vi "ScreenShots_Main_VIs.vi"(8 "error in":errorcluster, 9 "Bild Auswahl":T1[](array[typedef]), 10 "filename":string[](array[string]), 11 "Screenshots Pfad":path) -> (0 "error out":errorcluster, 3 "Screenshots Pfad out":path caption="Screenshots Pfad")   [LabVIEW 2020, in "Backup.lvlib"]
uses:
  Backup.lvlib
  Bildwechsel/Bild-Auswahl.ctl
  Bildwechsel/Bildwechsel.lvlib
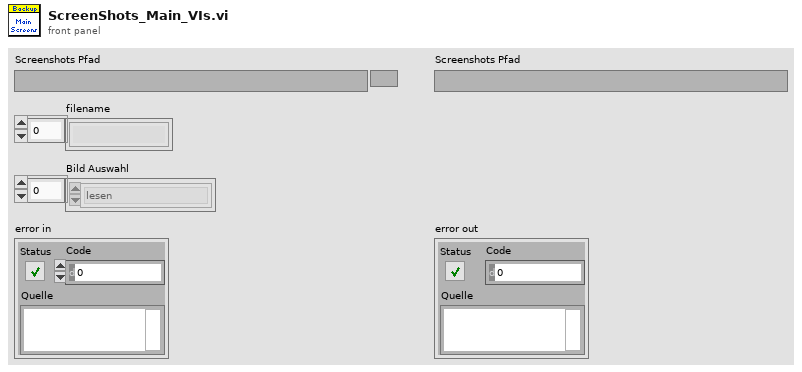
[diagram p1: front panel]
types:
  T1 = typedef "Bildwechsel.lvlib/Bild-Auswahl.ctl" = enum16{"lesen", "Initialisieren", "Beenden", "Grafik", "Anlagenübersicht", "Anlagengrenzwerte", "Log Konfig", "Gaszuordnung AO", "Erw. Konfiguration", "FT-IR  ", "Störmeldungen", "Störmeldepuffer", "Störmeldekonfig", "PNS Grenzwerte", "Statusübersicht", "Linearisierung", "ARN", "EPA Dichtheitstest", "FID", "PMA", "CalGas", "Lambda", "Interference", "Amium PNS", "EPA T90", "Interference N2O", "Scheduler", "Systemeinstellungen", "EPA Drift", "CAN Konfig"}
  T2 = typedef "imagedata.ctl" = cluster{"image type":i32, "image depth":i32, "image":u8[], "mask":u8[], "colors":u32[], "Rectangle":cluster{"left":i16, "top":i16, "right":i16, "bottom":i16}}
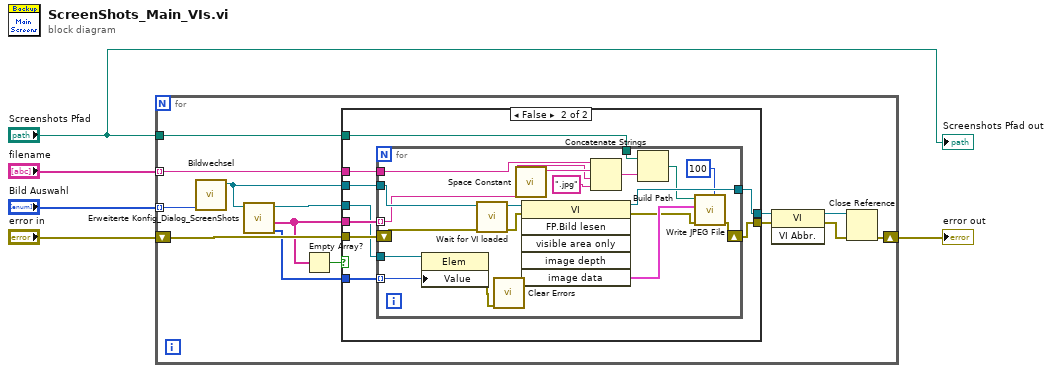
[diagram p0: block diagram]
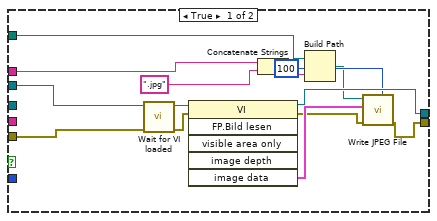
[diagram p2: hidden frame]
diagram:
  n1 = for {
    tunnel: "Screenshots Pfad" -> [w11]
    tunnel: "filename" -> [w12] mode=indexing
    shift-right: [w15] -> w5
    shift-left: "error in" -> [w13]
    tunnel: "Bild Auswahl" -> [w14] mode=indexing
    n2 = call "Bildwechsel.vi"("nächstes Bild"=w14) -> ("VI-Referenz neu"=w10:refnum<vi>)  [unwired: 9 in, 1 out]
    n3 = call "Erweiterte Konfig_Dialog_ScreenShots.vi"("VI-Referenz neu"=w10) -> ("Aktive Seiten"=w6:i32[], "Seitennamen"=w9:string[], "Elem Referenz"=w7:refnum<vi>)  [unwired: 8 in]
    n4 = Empty Array?(array=w9) -> (empty?=w8:bool)
    n5 = case shown="False" w8 {
      tunnel: [w33 w42] -> w19
      tunnel: [w32 w41] -> w18
      tunnel: w13 -> [w31 w40]
      tunnel: w12 -> [w30 w39]
      tunnel: w11 -> [w29 w38]
      tunnel: w10 -> [w28 w37]
      tunnel: w9 -> [_ w36]
      tunnel: w7 -> [_ w35]
      tunnel: w6 -> [_ w34]
      frame True {
        n6 = call "Wait for VI loaded.vi"("error in"=w31, "VI Referenz"=w28) -> ("error out"=w22:errorcluster, "VI Referenz out"=w23:refnum<vi>)  [unwired: 7 in, 1 out]
        n7 = invoke class="VI" method="FP.Bild lesen"(reference=w23, error in=w22) -> (reference out=w32:refnum<vi>, error out=w26:errorcluster, "image data"=w27:T2)  [unwired: 4 in, 3 out]
        n8 = Concatenate Strings(w30, ".jpg" ("String")) -> (w21:string)
        n9 = Build Path(base path=w29, name or relative path=w21) -> (appended path=w20:path)
        n10 = call <vilib>:"Write JPEG File.vi"("quality (80)"=100, "error in (no error)"=w26, "image data"=w27, "path to JPEG file"=w20) -> ("error out"=w33:errorcluster)  [unwired: 6 in, 1 out]
      }
      frame False {
        n11 = for {
          tunnel: [w60] -> w41
          shift-right: [w61] -> w42
          shift-left: w40 -> [w53]
          tunnel: w39 -> [w48]
          tunnel: w38 -> [w51]
          tunnel: w37 -> [w49]
          tunnel: w36 -> [w46] mode=indexing
          tunnel: w35 -> [w45]
          tunnel: w34 -> [w43] mode=indexing
          n12 = property class="Elem"(reference=w45, "Value"=w43) -> (error out=w44:errorcluster)  [unwired: 1 in, 1 out]
          n13 = call "Wait for VI loaded.vi"("error in"=w53, "VI Referenz"=w49) -> ("error out"=w54:errorcluster, "VI Referenz out"=w55:refnum<vi>)  [unwired: 7 in, 1 out]
          n14 = call <vilib>:"Clear Errors.vi"("error in (no error)"=w44) -> ()  [unwired: 5 in, 2 out]
          n15 = call <vilib>:"Space Constant.vi"() -> ("String"=w47:string)
          n16 = invoke class="VI" method="FP.Bild lesen"(reference=w55, error in=w54) -> (reference out=w60:refnum<vi>, error out=w58:errorcluster, "image data"=w59:T2)  [unwired: 4 in, 3 out]
          n17 = Concatenate Strings(w48, w47, w46, ".jpg" ("String")) -> (w52:string)
          n18 = Build Path(base path=w51, name or relative path=w52) -> (appended path=w50:path)
          n19 = call <vilib>:"Write JPEG File.vi"("quality (80)"=100, "error in (no error)"=w58, "image data"=w59, "path to JPEG file"=w50) -> ("error out"=w61:errorcluster)  [unwired: 6 in, 1 out]
        }
      }
    }
    n20 = invoke class="VI" method="VI Abbr."(reference=w18, error in=w19) -> (reference out=w17:refnum<vi>, error out=w16:errorcluster)  [unwired: 1 in, 1 out]
    n21 = Close Reference(reference=w17, error in (no error)=w16) -> (error out=w15:errorcluster)
  }
  "error out" <- w5
  "Screenshots Pfad out" <- "Screenshots Pfad"
